vi "configure.vi"(8 "error in (no error)":errorcluster, 11 "ScanModeMG091111IntrinsicImaging in":refnum<class "ImagingModeMG091111IntrinsicImaging.lvclass">) -> (0 "error out":errorcluster, 3 "ScanModeMG091111IntrinsicImaging out":refnum<class "ImagingModeMG091111IntrinsicImaging.lvclass">)   [LabVIEW 2010, in "ImagingModeMG091111IntrinsicImaging.lvclass"]
doc: "The dynamic dispatch version of this VI loads and displays the configuration file associated with the plug-in object. The user modify and save the configuration data."
uses:
  ImagingModeMG091111IntrinsicImaging.lvclass
  ImagingModeDL090923Scaffold/ImagingModeDL090923Scaffold/configuration_visibility_cluster.ctl
  ImagingModeDL090923Scaffold/ImagingModeDL090923Scaffold/component_configuration_visibility_cluster.ctl
  ImagingModeDL090923Scaffold/ImagingModeDL090923Scaffold/ImagingModeDL090923Scaffold.lvclass
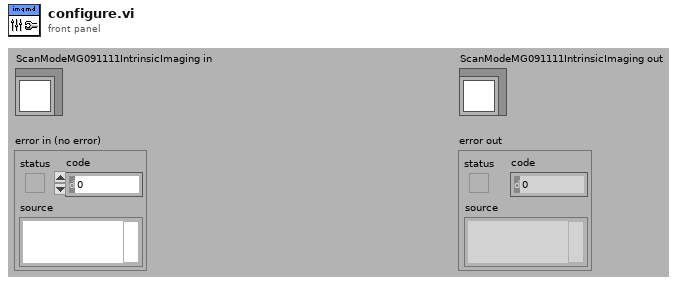
[diagram p1: front panel]
types:
  T1 = typedef "ImagingModeDL090923Scaffold.lvclass/configuration_visibility_cluster.ctl" = cluster{"Instrument":T2, "Trajectory":T2, "ScanHead":T2, "DAQ":T2, "ImageAssembler":T2, "DataCollection":T2, "Display":T2, "Analyser":T2, "Stimulator":T2, "enable Trajectory-to-ImageAssembler adapter":bool}
  T2 = typedef "ImagingModeDL090923Scaffold.lvclass/component_configuration_visibility_cluster.ctl" = cluster{"enable":bool, "enable adapter":bool}
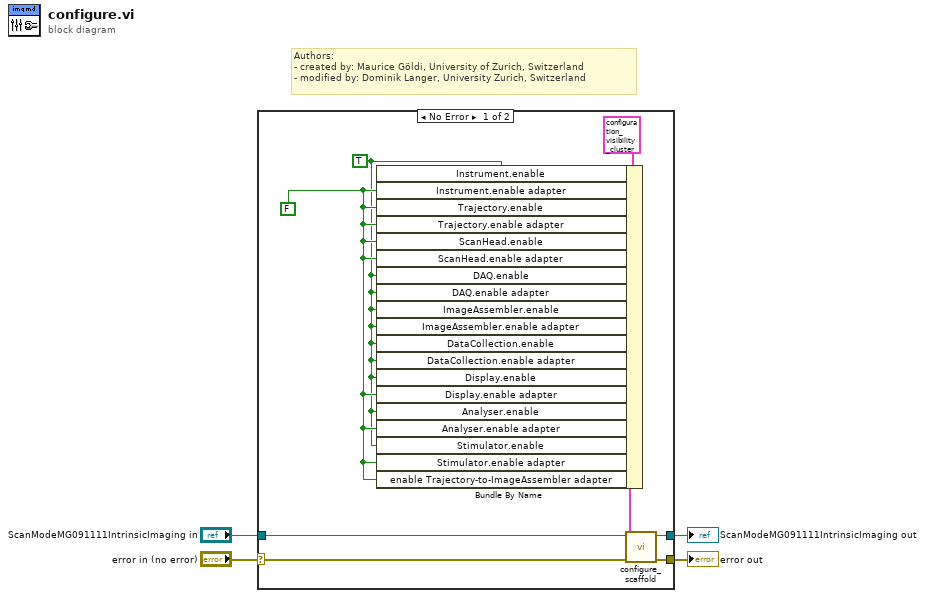
[diagram p0: block diagram]
diagram:
  # "Authors: \n- created by: Maurice Göldi, University of Zurich, Switzerland\n- modified by: Dominik Langer, University Zurich, Switzerland"
  n1 = case shown="No Error" "error in (no error)" {
    selector: "error in (no error)" -> [w9 w13]
    tunnel: [w12 w13] -> w4
    tunnel: [w11 w14] -> w3
    tunnel: "ScanModeMG091111IntrinsicImaging in" -> [w10 w14]
    frame No Error {
      w6 = TRUE
      w7 = FALSE
      n2 = Bundle By Name(cluster=T1 {"Instrument"={"enable"=FALSE, "enable adapter"=FALSE}, "Trajectory"={"enable"=FALSE, "enable adapter"=FALSE}, "ScanHead"={"enable"=FALSE, "enable adapter"=FALSE}, "DAQ"={"enable"=FALSE, "enable adapter"=FALSE}, "ImageAssembler"={"enable"=FALSE, "enable adapter"=FALSE}, "DataCollection"={"enable"=FALSE, "enable adapter"=FALSE}, "Display"={"enable"=FALSE, "enable adapter"=FALSE}, "Analyser"={"enable"=FALSE, "enable adapter"=FALSE}, "Stimulator"={"enable"=FALSE, "enable adapter"=FALSE}, "enable Trajectory-to-ImageAssembler adapter"=FALSE} ("visibilities"), "Instrument.enable"=w6, "Instrument.enable adapter"=w7, "Trajectory.enable"=w7, "Trajectory.enable adapter"=w7, "ScanHead.enable"=w7, "ScanHead.enable adapter"=w7, "DAQ.enable"=w6, "DAQ.enable adapter"=w6, "ImageAssembler.enable"=w6, "ImageAssembler.enable adapter"=w6, "DataCollection.enable"=w6, "DataCollection.enable adapter"=w6, "Display.enable"=w6, "Display.enable adapter"=w7, "Analyser.enable"=w6, "Analyser.enable adapter"=w7, "Stimulator.enable"=w6, "Stimulator.enable adapter"=w7, "enable Trajectory-to-ImageAssembler adapter"=w7) -> (w8:T1)
      n3 = call-dynamic "configure_scaffold.vi"("error in (no error)"=w9, "visibilities"=w8, "ScanModeDL090923Scaffold in"=w10) -> ("error out"=w12:errorcluster, "ScanModeDL090923Scaffold out"=w11:refnum<class "ImagingModeMG091111IntrinsicImaging.lvclass">)  [unwired: 7 in]
    }
    frame Error {
    }
  }
  "error out" <- w4
  "ScanModeMG091111IntrinsicImaging out" <- w3
